vi "Create Buss Park.vi"(6 "sample rate":dbl=1000.0 format="%#_6p", 7 "OVS":u8=16, 8 "error in (no error)":errorcluster) -> (0 "error out":errorcluster, 3 "Digital Waveform Graph":digitalwaveform(graph))   [LabVIEW 2013]
uses:
  <vilib>/Waveform/DWDTOps.llb/Digital Pattern Generator (Single Value).vi
  <vilib>/Waveform/DWDTOps.llb/DWDT Append Digital Samples.vi
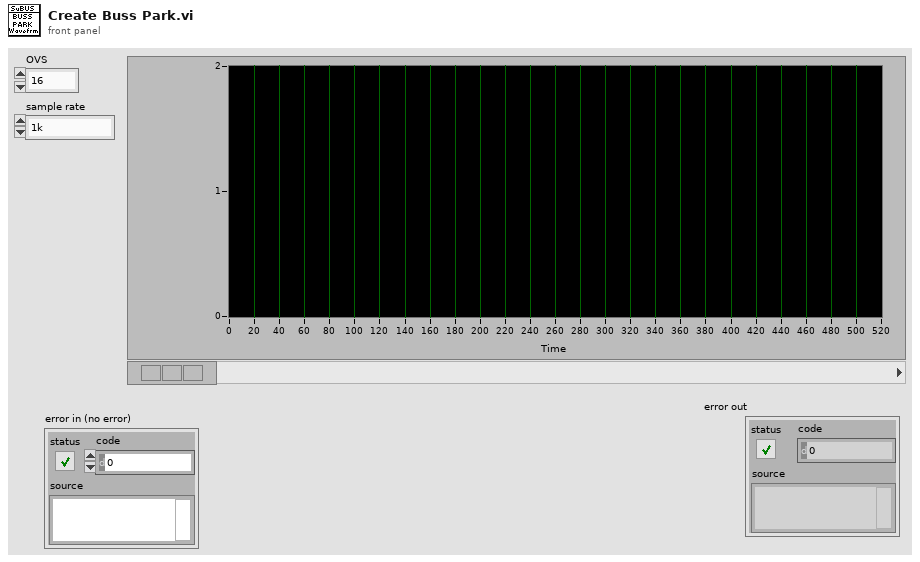
[diagram p1: front panel]
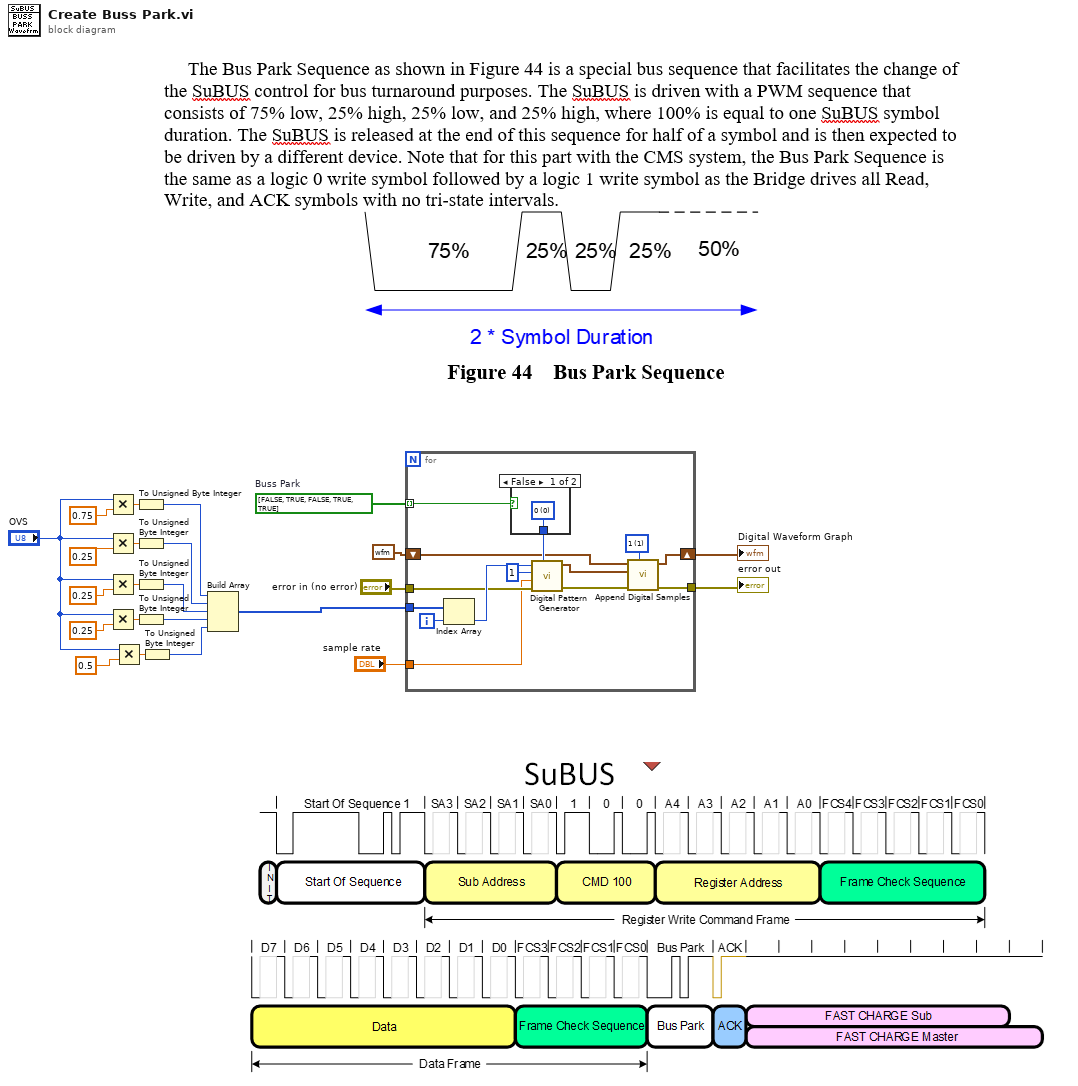
[diagram p0: block diagram]
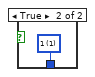
[diagram p2: hidden frame]
diagram:
  w10 = bool[] [FALSE, TRUE, FALSE, TRUE, TRUE]  # Buss Park
  n1 = Multiply(x="OVS", y=0.75) -> (x*y=w23:dbl)
  n2 = Multiply(x="OVS", y=0.25) -> (x*y=w21:dbl)
  n3 = Multiply(x="OVS", y=0.25) -> (x*y=w19:dbl)
  n4 = Multiply(x="OVS", y=0.25) -> (x*y=w17:dbl)
  n5 = Multiply(x="OVS", y=0.5) -> (x*y=w4:dbl)
  n6 = To Unsigned Byte Integer(number=w23) -> (unsigned 8bit integer=w15:u8)
  n7 = To Unsigned Byte Integer(number=w21) -> (unsigned 8bit integer=w14:u8)
  n8 = To Unsigned Byte Integer(number=w19) -> (unsigned 8bit integer=w13:u8)
  n9 = To Unsigned Byte Integer(number=w17) -> (unsigned 8bit integer=w12:u8)
  n10 = To Unsigned Byte Integer(number=w4) -> (unsigned 8bit integer=w1:u8)
  n11 = Build Array(w15, w14, w13, w12, w1) -> (w11:u8[])
  n12 = for {
    tunnel: w11 -> [w37]
    tunnel: w10 -> [w34] mode=indexing
    shift-right: [w28] -> w6
    shift-left: digitalwaveform {"t0"=timestamp(0 s since 1904-01-01), "dt"=0.0, "Y"={"transitions"=[], "data"=[]}} ("digital waveform out") -> [w27]
    tunnel: "error in (no error)" -> [w26]
    tunnel: [w25] -> w7
    tunnel: "sample rate" -> [w24]
    i -> [w36]
    w31 = u8 1 items=["0", "1", "Z", "L", "H", "X", "T", "V"] ("default value")
    n13 = Index Array(array=w37, index=w36) -> (element=w32:u8)
    n14 = case shown="False" w34 {
      tunnel: [w38 w39] -> w33
      frame False {
        w38 = u8 0 items=["0", "1", "Z", "L", "H", "X", "T", "V"] ("value")
      }
      frame True {
        w39 = u8 1 items=["0", "1", "Z", "L", "H", "X", "T", "V"] ("value")
      }
    }
    n15 = call-poly <vilib>:"Digital Pattern Generator.vi"("value"=w33, "error in (no error)"=w26, "sample rate"=w24, "number of signals"=u32 1, "number of samples"=w32) -> ("error out"=w30:errorcluster, "digital waveform"=w29:digitalwaveform)  [unwired: 5 in]
    n16 = call-poly <vilib>:"Append Digital Samples.vi"("default value"=w31, "error in (no error)"=w30, "digital waveform B"=w29, "digital waveform A"=w27) -> ("error out"=w25:errorcluster, "digital waveform out"=w28:digitalwaveform)  [unwired: 6 in]
  }
  "error out" <- w7
  "Digital Waveform Graph" <- w6
